vi "Tree.vi"() -> ()   [LabVIEW 2016, in "Data.ITX.lvclass"]
uses:
  Data.ITX.lvclass
  Data/Data.lvclass
  Data.DAT/Data.DAT.lvclass
  Data.TDMS/Data.TDMS.lvclass
  Data.HDF5/Data.HDF5.lvclass
  Data/Typedefs/Type--enum.ctl
  Data/Typedefs/Dictionary--cluster.ctl
panel:
  in  "Append? [F]":bool
  in  "File Type 2":T1
  in  "error in (no error)":errorcluster
  in  "Notes 2":string
  in  "Data (Dictionary) 2":T2[](array[typedef])
  in  "path":path
  out "path out":path
  out "Data (Dictionary)":T2[](array[typedef])
  out "Notes":string
  out "error out":errorcluster
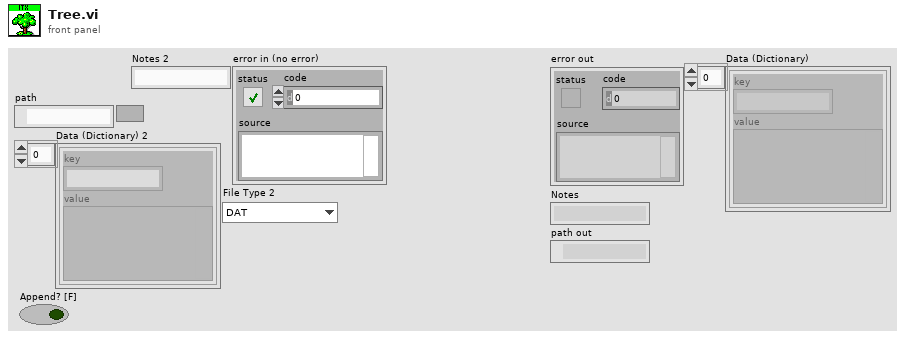
[diagram p1: front panel]
types:
  T1 = typedef "Data.lvclass/Type--enum.ctl" = enum16{"DAT", "ITX", "HDF5", "TDMS", "VI"}
  T2 = typedef "Data.lvclass/Dictionary--cluster.ctl" = cluster{"key":string, "value":variant}
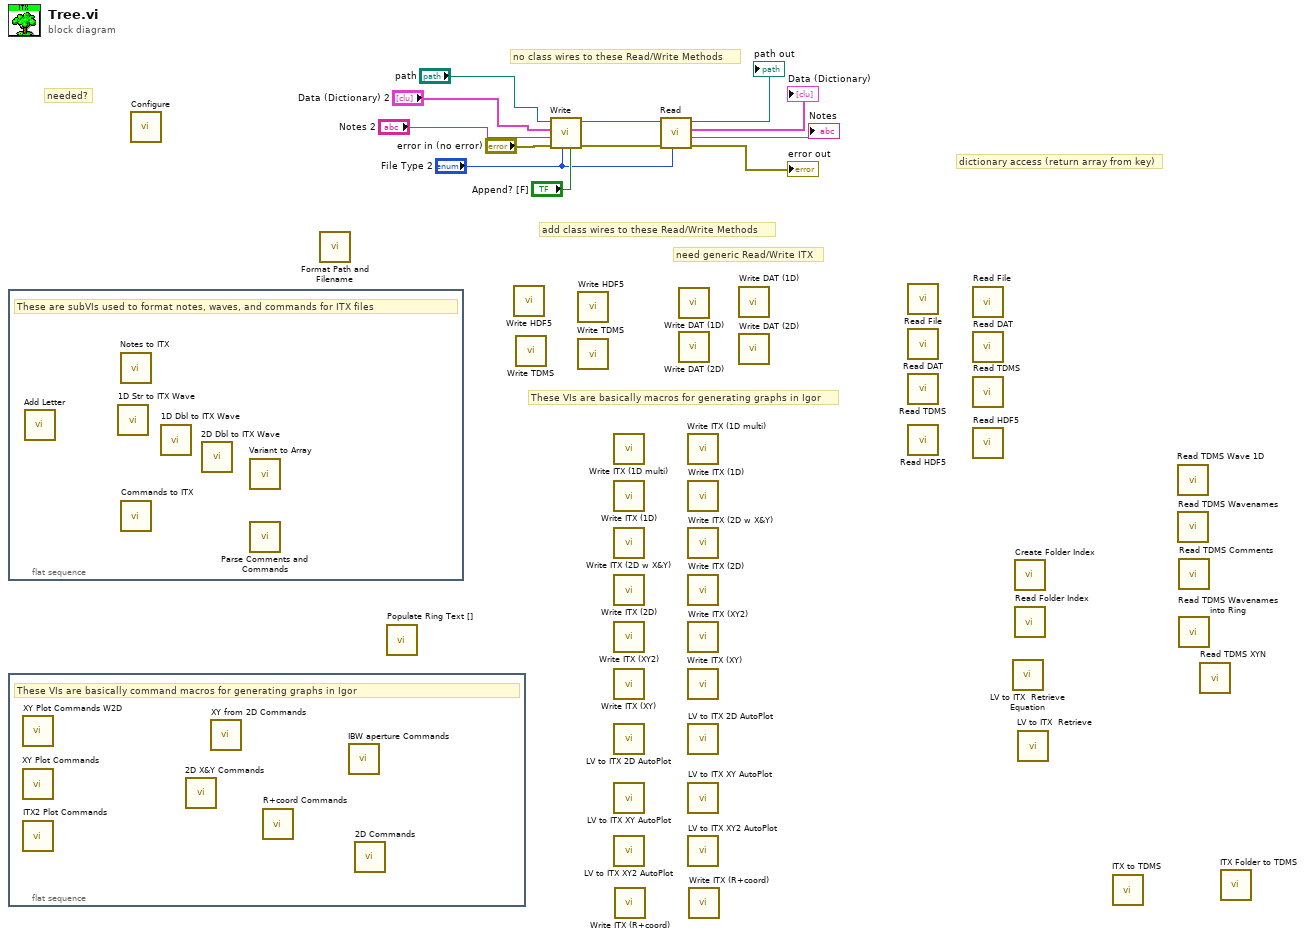
[diagram p0: block diagram]
diagram:
  # "needed?"
  # "These VIs are basically macros for generating graphs in Igor"
  # "need generic Read/Write ITX"
  # "dictionary access (return array from key)"
  # "no class wires to these Read/Write Methods"
  # "add class wires to these Read/Write Methods"
  n1 = flat-sequence {
    frame #0 {
      # "These are subVIs used to format notes, waves, and commands for ITX files"
      n2 = call "Add Letter.vi"() -> ()  [unwired: 1 in, 1 out]
      n3 = call "1D Str to ITX Wave.vi"() -> ()  [unwired: 2 in, 1 out]
      n4 = call "Notes to ITX.vi"() -> ()  [unwired: 1 in, 1 out]
      n5 = call "Commands to ITX.vi"() -> ()  [unwired: 1 in, 1 out]
      n6 = call "1D Dbl to ITX Wave.vi"() -> ()  [unwired: 2 in, 1 out]
      n7 = call "2D Dbl to ITX Wave.vi"() -> ()  [unwired: 2 in, 1 out]
      n8 = call "Variant to Array.vi"() -> ()  [unwired: 9 in, 3 out]
      n9 = call "Parse Comments and Commands.vi"() -> ()  [unwired: 2 in, 2 out]
    }
  }
  n10 = flat-sequence {
    frame #0 {
      # "These VIs are basically command macros for generating graphs in Igor"
      n11 = call "XY Plot Commands W2D.vi"() -> ()  [unwired: 5 in, 1 out]
      n12 = call "XY Plot Commands.vi"() -> ()  [unwired: 6 in, 1 out]
      n13 = call "ITX2 Plot Commands.vi"() -> ()  [unwired: 6 in, 1 out]
      n14 = call "2D X&Y Commands.vi"() -> ()  [unwired: 10 in, 2 out]
      n15 = call "XY from 2D Commands.vi"() -> ()  [unwired: 2 in, 1 out]
      n16 = call "R+coord Commands.vi"() -> ()  [unwired: 15 in, 1 out]
      n17 = call "IBW aperture Commands.vi"() -> ()  [unwired: 4 in, 1 out]
      n18 = call "2D Commands.vi"() -> ()  [unwired: 15 in, 1 out]
    }
  }
  n19 = call-dynamic "Configure.vi"() -> ()  [unwired: 10 in, 2 out]
  n20 = call "Format Path and Filename.vi"() -> ()  [unwired: 9 in, 3 out]
  n21 = call "Populate Ring Text [].vi"() -> ()  [unwired: 11 in, 1 out]
  n22 = call "Write HDF5.vi"() -> ()  [unwired: 9 in, 3 out]
  n23 = call "Write TDMS.vi"() -> ()  [unwired: 9 in, 3 out]
  n24 = call "Write.vi"("Append? [F]"="Append? [F]", "File Type"="File Type 2", "error in (no error)"="error in (no error)", "Notes"="Notes 2", "Data (Dictionary)"="Data (Dictionary) 2", "path"="path") -> ("error out"=w8:errorcluster, "path out"=w9:path)  [unwired: 4 in]
  n25 = call "Write HDF5.vi"() -> ()  [unwired: 9 in, 3 out]
  n26 = call "Write TDMS.vi"() -> ()  [unwired: 9 in, 3 out]
  n27 = call "Write ITX (1D multi).vi"() -> ()  [unwired: 12 in]
  n28 = call "Write ITX (1D).vi"() -> ()  [unwired: 12 in]
  n29 = call "Write ITX (2D w X&Y).vi"() -> ()  [unwired: 11 in, 1 out]
  n30 = call "Write ITX (2D).vi"() -> ()  [unwired: 12 in]
  n31 = call "Write ITX (XY2).vi"() -> ()  [unwired: 11 in, 1 out]
  n32 = call "Write ITX (XY).vi"() -> ()  [unwired: 11 in, 1 out]
  n33 = call "LV to ITX 2D AutoPlot.vi"() -> ()  [unwired: 9 in, 3 out]
  n34 = call "LV to ITX XY AutoPlot.vi"() -> ()  [unwired: 9 in, 3 out]
  n35 = call "LV to ITX XY2 AutoPlot.vi"() -> ()  [unwired: 9 in, 3 out]
  n36 = call "Write ITX (R+coord).vi"() -> ()  [unwired: 12 in]
  n37 = call "Read.vi"("File Type"="File Type 2", "error in (no error)"=w8, "path"=w9) -> ("error out"=→"error out":errorcluster, "Notes"=→"Notes":string, "Data (Dictionary)"=→"Data (Dictionary)":T2[], "path out"=→"path out":path)  [unwired: 5 in]
  n38 = call "Write DAT (1D).vi"() -> ()  [unwired: 10 in, 2 out]
  n39 = call "Write DAT (2D).vi"() -> ()  [unwired: 10 in, 2 out]
  n40 = call "Write ITX (1D multi).vi"() -> ()  [unwired: 12 in]
  n41 = call "Write ITX (1D).vi"() -> ()  [unwired: 12 in]
  n42 = call "Write ITX (2D w X&Y).vi"() -> ()  [unwired: 11 in, 1 out]
  n43 = call "Write ITX (2D).vi"() -> ()  [unwired: 12 in]
  n44 = call "Write ITX (XY2).vi"() -> ()  [unwired: 11 in, 1 out]
  n45 = call "Write ITX (XY).vi"() -> ()  [unwired: 11 in, 1 out]
  n46 = call "LV to ITX 2D AutoPlot.vi"() -> ()  [unwired: 9 in, 3 out]
  n47 = call "LV to ITX XY AutoPlot.vi"() -> ()  [unwired: 9 in, 3 out]
  n48 = call "LV to ITX XY2 AutoPlot.vi"() -> ()  [unwired: 9 in, 3 out]
  n49 = call "Write ITX (R+coord).vi"() -> ()  [unwired: 12 in]
  n50 = call "Write DAT (1D).vi"() -> ()  [unwired: 10 in, 2 out]
  n51 = call "Write DAT (2D).vi"() -> ()  [unwired: 10 in, 2 out]
  n52 = call-dynamic "Read File.vi"() -> ()  [unwired: 10 in, 2 out]
  n53 = call "Read DAT.vi"() -> ()  [unwired: 9 in, 3 out]
  n54 = call "Read TDMS.vi"() -> ()  [unwired: 8 in, 4 out]
  n55 = call "Read HDF5.vi"() -> ()  [unwired: 8 in, 4 out]
  n56 = call-dynamic "Read File.vi"() -> ()  [unwired: 10 in, 2 out]
  n57 = call "Read DAT.vi"() -> ()  [unwired: 9 in, 3 out]
  n58 = call "Read TDMS.vi"() -> ()  [unwired: 8 in, 4 out]
  n59 = call "Read HDF5.vi"() -> ()  [unwired: 8 in, 4 out]
  n60 = call "LV to ITX  Retrieve Equation.vi"() -> ()  [unwired: 11 in, 5 out]
  n61 = call "Create Folder Index.vi"() -> ()  [unwired: 11 in, 1 out]
  n62 = call "Read Folder Index.vi"() -> ()  [unwired: 10 in, 2 out]
  n63 = call "LV to ITX  Retrieve.vi"() -> ()  [unwired: 11 in, 5 out]
  n64 = call "ITX to TDMS.vi"() -> ()  [unwired: 10 in, 2 out]
  n65 = call "Read TDMS Wave 1D.vi"() -> ()  [unwired: 9 in, 3 out]
  n66 = call "Read TDMS Wavenames.vi"() -> ()  [unwired: 9 in, 3 out]
  n67 = call "Read TDMS Comments.vi"() -> ()  [unwired: 9 in, 3 out]
  n68 = call "Read TDMS Wavenames into Ring.vi"() -> ()  [unwired: 10 in, 2 out]
  n69 = call "Read TDMS XYN.vi"() -> ()  [unwired: 8 in, 4 out]
  n70 = call "ITX Folder to TDMS.vi"() -> ()  [unwired: 10 in, 2 out]
